vi "ReadLogStartNode.vi"(8 "Error In":errorcluster, 11 "Keithley2602 Node In":refnum<k20>) -> (0 "Error Out":errorcluster, 2 "Log Start Configuration":T1, 3 "Keithley2602 Node Out":refnum<k20>)   [LabVIEW 2013]
uses:
  LogStartConfiguration.ctl
  LogStartTriggerType.ctl
  LogDigitalIOTriggerEdge.ctl
  <vilib>/xml/NI_XML.lvlib
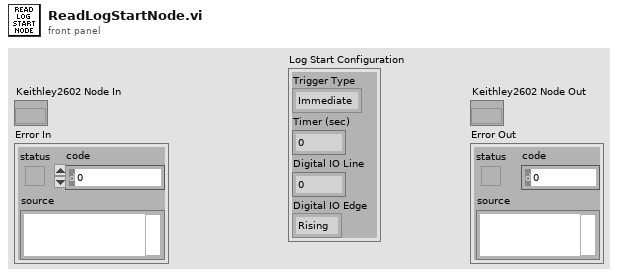
[diagram p1: front panel]
types:
  T1 = typedef "LogStartConfiguration.ctl" = cluster{"Trigger Type":T2, "Timer (sec)":dbl, "Digital IO Line":u8, "Digital IO Edge":T3}
  T2 = typedef "LogStartTriggerType.ctl" = enum16{"Immediate", "User", "Timer", "Digital IO"}
  T3 = typedef "LogDigitalIOTriggerEdge.ctl" = enum16{"Rising", "Falling"}
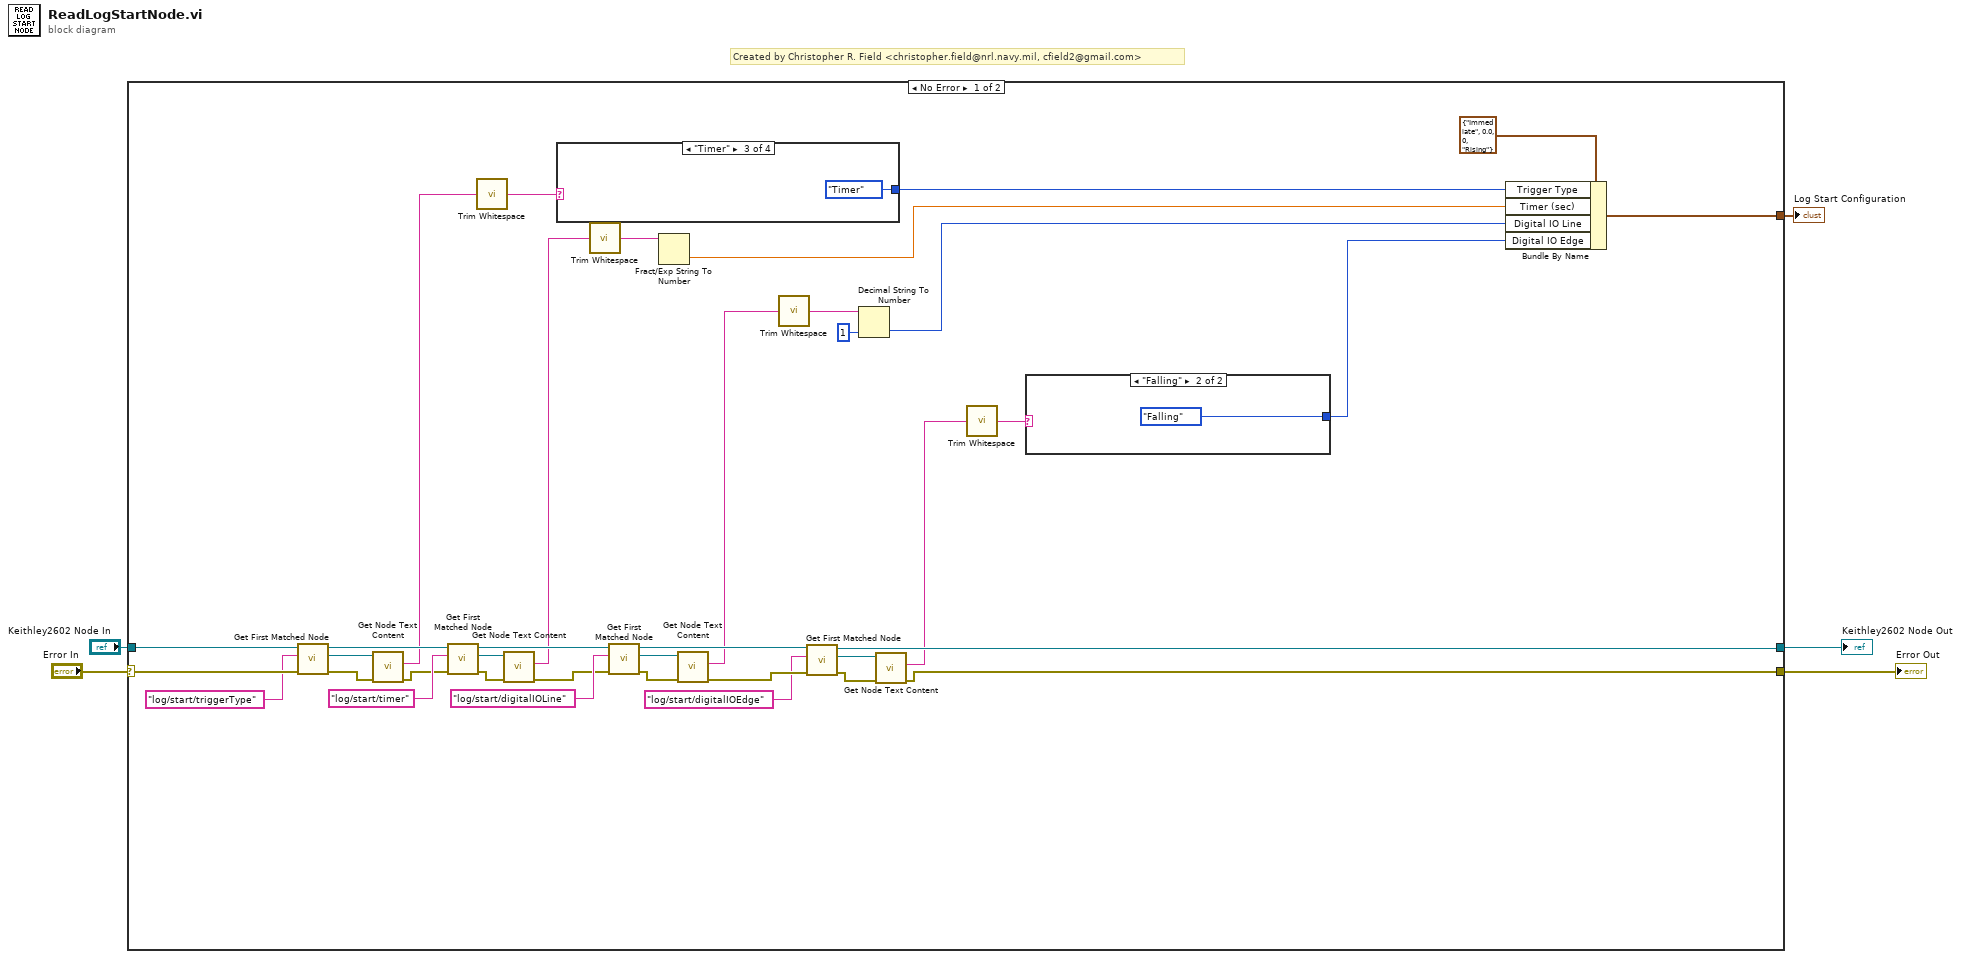
[diagram p0: block diagram]
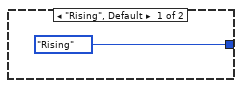
[diagram p2: hidden frame]
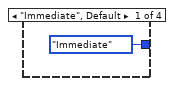
[diagram p3: hidden frame]
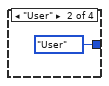
[diagram p4: hidden frame]
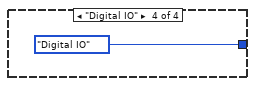
[diagram p5: hidden frame]
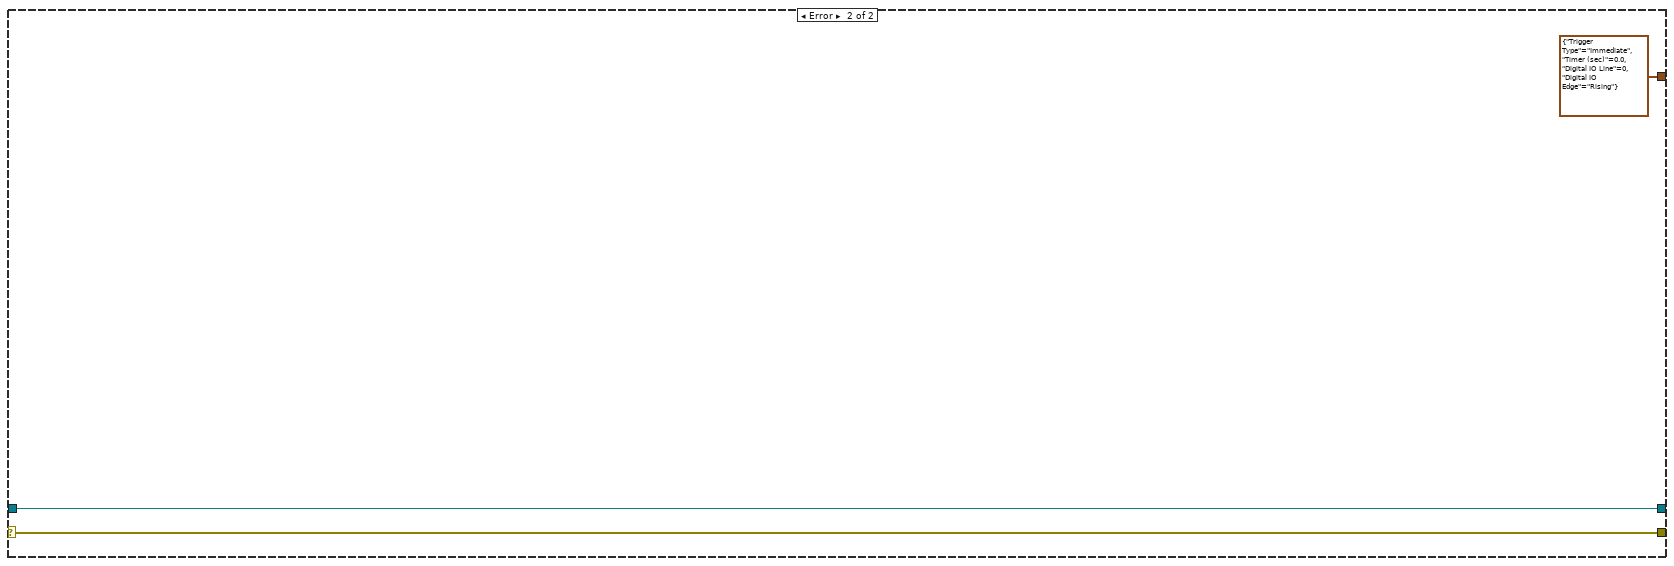
[diagram p6: hidden frame]
diagram:
  # "Created by Christopher R. Field <christopher.field@nrl.navy.mil, cfield2@gmail.com>"
  n1 = case shown="No Error" "Error In" {
    selector: "Error In" -> [w40 w50]
    tunnel: "Keithley2602 Node In" -> [w41 w51]
    tunnel: [w16 w51] -> w3
    tunnel: [w15 w50] -> w2
    tunnel: [w14 T1 {"Trigger Type"=enum."Immediate", "Timer (sec)"=0.0, "Digital IO Line"=0, "Digital IO Edge"=enum."Rising"} ("Log Start Configuration")] -> w1
    frame No Error {
      n2 = call <vilib>:"Get First Matched Node.vi"("error in (no error)"=w40, "XPath expression"="log/start/triggerType", "node in"=w41) -> ("error out"=w37:errorcluster, "node result"=w38:refnum<k20>, "node out"=w34:refnum<k20>)  [unwired: 6 in]
      n3 = call <vilib>:"Get Node Text Content.vi"("error in (no error)"=w37, "node in"=w38) -> ("error out"=w33:errorcluster, "node text"=w12:string)  [unwired: 7 in, 1 out]
      n4 = call <vilib>:"Get First Matched Node.vi"("error in (no error)"=w33, "XPath expression"="log/start/timer", "node in"=w34) -> ("error out"=w31:errorcluster, "node result"=w32:refnum<k20>, "node out"=w28:refnum<k20>)  [unwired: 6 in]
      n5 = call <vilib>:"Trim Whitespace.vi"("string"=w12) -> ("trimmed string"=w13:string)  [unwired: 1 in]
      n6 = call <vilib>:"Get Node Text Content.vi"("error in (no error)"=w31, "node in"=w32) -> ("error out"=w27:errorcluster, "node text"=w10:string)  [unwired: 7 in, 1 out]
      n7 = case shown="\"Timer\"" w13 {
        tunnel: [LogStartTriggerType."Immediate" ("Trigger Type") LogStartTriggerType."User" ("Trigger Type") LogStartTriggerType."Timer" ("Trigger Type") LogStartTriggerType."Digital IO" ("Trigger Type")] -> w36
        frame "Immediate", Default {
        }
        frame "User" {
        }
        frame "Timer" {
        }
        frame "Digital IO" {
        }
      }
      n8 = call <vilib>:"Trim Whitespace.vi"("string"=w10) -> ("trimmed string"=w11:string)  [unwired: 1 in]
      n9 = call <vilib>:"Get First Matched Node.vi"("error in (no error)"=w27, "XPath expression"="log/start/digitalIOLine", "node in"=w28) -> ("error out"=w25:errorcluster, "node result"=w26:refnum<k20>, "node out"=w20:refnum<k20>)  [unwired: 6 in]
      n10 = Fract/Exp String To Number(string=w11) -> (number=w30:dbl)  [unwired: 3 in, 1 out]
      n11 = call <vilib>:"Get Node Text Content.vi"("error in (no error)"=w25, "node in"=w26) -> ("error out"=w19:errorcluster, "node text"=w8:string)  [unwired: 7 in, 1 out]
      n12 = call <vilib>:"Trim Whitespace.vi"("string"=w8) -> ("trimmed string"=w9:string)  [unwired: 1 in]
      n13 = call <vilib>:"Get First Matched Node.vi"("error in (no error)"=w19, "XPath expression"="log/start/digitalIOEdge", "node in"=w20) -> ("error out"=w21:errorcluster, "node result"=w22:refnum<k20>, "node out"=w16:refnum<k20>)  [unwired: 6 in]
      n14 = Decimal String To Number(string=w9, default (0L)=u32 1 ("default (0 I32)")) -> (number=w23:u32)  [unwired: 1 in, 1 out]
      n15 = call <vilib>:"Get Node Text Content.vi"("error in (no error)"=w21, "node in"=w22) -> ("error out"=w15:errorcluster, "node text"=w6:string)  [unwired: 7 in, 1 out]
      n16 = call <vilib>:"Trim Whitespace.vi"("string"=w6) -> ("trimmed string"=w7:string)  [unwired: 1 in]
      n17 = case shown="\"Falling\"" w7 {
        tunnel: [LogDigitalIOTriggerEdge."Rising" ("Digital IO Edge") LogDigitalIOTriggerEdge."Falling" ("Digital IO Edge")] -> w17
        frame "Rising", Default {
        }
        frame "Falling" {
        }
      }
      n18 = Bundle By Name(cluster=T1 {"Trigger Type"=enum."Immediate", "Timer (sec)"=0.0, "Digital IO Line"=0, "Digital IO Edge"=enum."Rising"} ("Log Start Configuration"), "Trigger Type"=w36, "Timer (sec)"=w30, "Digital IO Line"=w23, "Digital IO Edge"=w17) -> (w14:T1)
    }
    frame Error {
    }
  }
  "Keithley2602 Node Out" <- w3
  "Error Out" <- w2
  "Log Start Configuration" <- w1
